vi "Read FITS Header.vi"(0 "Input File:":path=path "", 11 "error in":errorcluster) -> (1 "Header length":i32, 2 "Header":string, 3 "File Read:":path, 4 "Header Lines":i32, 8 "NAXIS1":i32, 10 "NAXIS2":i32, 12 "SIMPLE":string, 13 "BITPIX":i32, 14 "NAXIS":i32, 15 "error out":errorcluster)   [LabVIEW 2024]
uses:
  <vilib>/Utility/error.llb/whitespace.ctl
  <vilib>/Utility/error.llb/Trim Whitespace One-Sided.vi
panel:
  out "Characters":i32
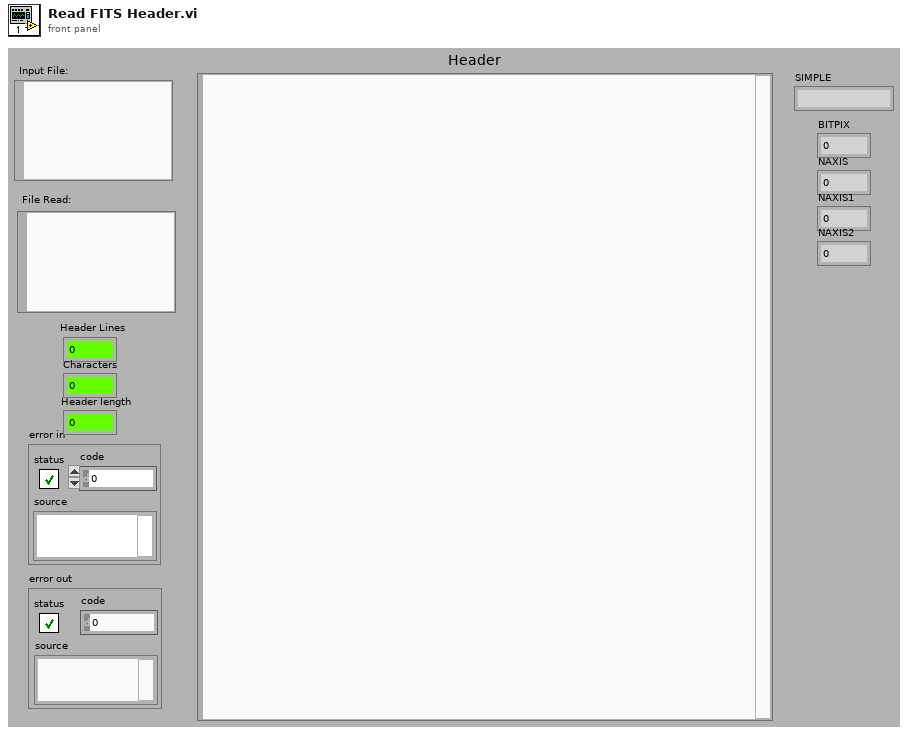
[diagram p1: front panel]
types:
  T1 = typedef "whitespace.ctl" = u16
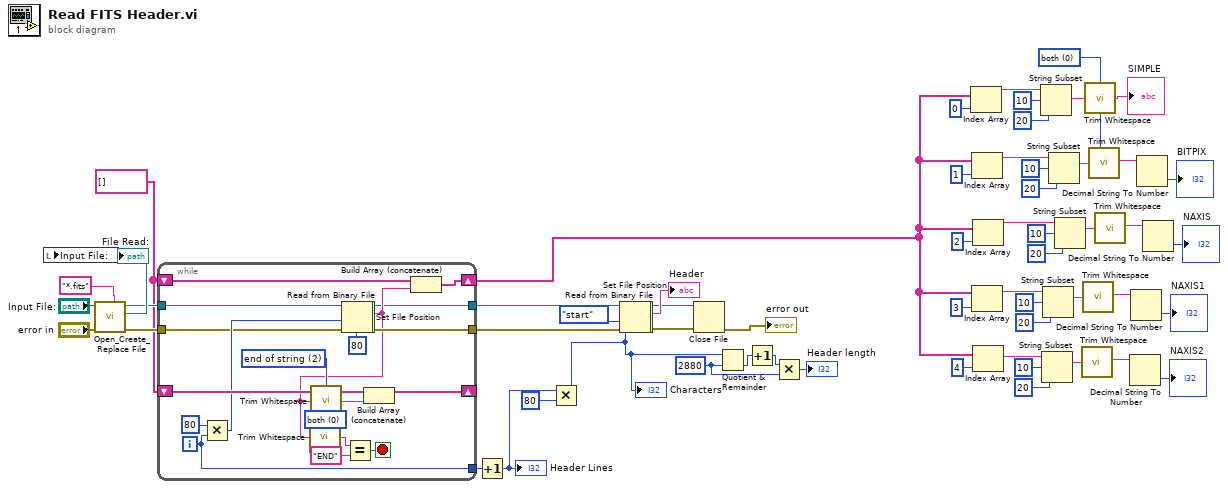
[diagram p0: block diagram]
diagram:
  w4 = string[] []
  w14 = 2880 ("y")
  w44 = T1 0 items=["both", "start of string", "end of string"] ("location (both)")
  n1 = call <vilib>:"Open_Create_Replace File.vi"("pattern"="*.fits", "error in (no error)"="error in", "file path"="Input File:") -> ("error out"=w19:errorcluster, "new file path"=w18:path, "refnum"=w7:refnum<file>)  [unwired: 5 in, 1 out]
  "File Read:" <- w18
  n2 = local write "Input File:"(w18) -> ()
  n3 = while {
    shift-right: [w76] -> _
    shift-left: w4 -> [w75]
    tunnel: [w73] -> w60
    shift-right: [w65] -> w5
    shift-left: w4 -> [w72]
    tunnel: [w70] -> w8
    tunnel: w19 -> [w67]
    tunnel: [w64] -> w9
    tunnel: w7 -> [w63]
    i -> [w73]
    stop <- w81 stop-if-true
    w77 = T1 2 items=["both", "start of string", "end of string"] ("location (both)")
    w78 = T1 0 items=["both", "start of string", "end of string"] ("location (both)")
    n4 = Multiply(x=80, y=w73) -> (x*y=w69:i32)
    n5 = Set File Position(offset (in bytes) (0)=w69, refnum=w63, error in=w67) -> (refnum out=w62:refnum<file>, error out=w61:errorcluster)  [unwired: 1 in]
    n6 = Read from Binary File(8:w61, 10:80 ("[max characters per line]  (no limit:0)"), 11:w62) -> (0:w70:errorcluster, 2:w66:string, 3:w64:refnum<file>)  [unwired: 3 in, 1 out]
    n7 = call <vilib>:"Trim Whitespace.vi"("string"=w66, "location (both)"=w78) -> ("trimmed string"=w79:string)
    n8 = call <vilib>:"Trim Whitespace.vi"("string"=w66, "location (both)"=w77) -> ("trimmed string"=w74:string)
    n9 = Equal?(x=w79, y="END") -> (x = y?=w81:bool)
    n10 = Build Array (concatenate)(w75, w74) -> (w76:string[])
    n11 = Build Array (concatenate)(w72, w66) -> (w65:string[])
  }
  n12 = Increment(x=w60) -> (x+1=w17:i32)
  "Header Lines" <- w17
  n13 = Multiply(x=w17, y=80) -> (x*y=w6:i32)
  "Characters" <- w6
  n14 = Set File Position(refnum=w9, from (0:start)=enum16{"start", "end", "current"}."start" ("pos mode (0:2)"), error in=w8) -> (refnum out=w2:refnum<file>, error out=w1:errorcluster)  [unwired: 1 in]
  n15 = Read from Binary File(8:w1, 10:w6, 11:w2) -> (0:w20:errorcluster, 2:→"Header":string, 3:w10:refnum<file>)  [unwired: 3 in, 1 out]
  n16 = Close File(refnum=w10, error in=w20) -> (error out=→"error out":errorcluster)  [unwired: 1 out]
  n17 = Quotient & Remainder(x=w6, y=w14) -> (floor(x/y)=w12:i32)  [unwired: 1 out]
  n18 = Increment(x=w12) -> (x+1=w15:i32)
  n19 = Multiply(x=w15, y=w14) -> (x*y=→"Header length":i32)
  n20 = Index Array(array=w5, index=0) -> (element=w52:string)
  n21 = Index Array(array=w5, index=1) -> (element=w45:string)
  n22 = Index Array(array=w5, index=3) -> (element=w29:string)
  n23 = Index Array(array=w5, index=2) -> (element=w35:string)
  n24 = Index Array(array=w5, index=4) -> (element=w23:string)
  n25 = String Subset(string=w52, offset (0)=10, length (rest)=20 ("length (rest)")) -> (substring=w49:string)
  n26 = String Subset(string=w23, offset (0)=10, length (rest)=20 ("length (rest)")) -> (substring=w26:string)
  n27 = String Subset(string=w29, offset (0)=10, length (rest)=20 ("length (rest)")) -> (substring=w32:string)
  n28 = String Subset(string=w45, offset (0)=10, length (rest)=20 ("length (rest)")) -> (substring=w43:string)
  n29 = String Subset(string=w35, offset (0)=10, length (rest)=20 ("length (rest)")) -> (substring=w38:string)
  n30 = call <vilib>:"Trim Whitespace.vi"("string"=w26) -> ("trimmed string"=w25:string)  [unwired: 1 in]
  n31 = call <vilib>:"Trim Whitespace.vi"("string"=w32) -> ("trimmed string"=w31:string)  [unwired: 1 in]
  n32 = call <vilib>:"Trim Whitespace.vi"("string"=w49, "location (both)"=w44) -> ("trimmed string"=→"SIMPLE":string)
  n33 = call <vilib>:"Trim Whitespace.vi"("string"=w43, "location (both)"=w44) -> ("trimmed string"=w42:string)
  n34 = call <vilib>:"Trim Whitespace.vi"("string"=w38) -> ("trimmed string"=w37:string)  [unwired: 1 in]
  n35 = Decimal String To Number(string=w25) -> (number=→"NAXIS2":i32)  [unwired: 2 in, 1 out]
  n36 = Decimal String To Number(string=w31) -> (number=→"NAXIS1":i32)  [unwired: 2 in, 1 out]
  n37 = Decimal String To Number(string=w42) -> (number=→"BITPIX":i32)  [unwired: 2 in, 1 out]
  n38 = Decimal String To Number(string=w37) -> (number=→"NAXIS":i32)  [unwired: 2 in, 1 out]
